vi "GetDescendants.vi"(8 "error in":errorcluster, 11 "node in":refnum<data-value>) -> (0 "error out":errorcluster, 3 "descendants":refnum<data-value>[](array[refnum]))   [LabVIEW 2023, in "CEF.lvlib" / "CEF_Node.lvclass"]
doc: "Copyright 2017 National Instruments Corporation\n\nLicensed under the Apache License, Version 2.0 (the \"License\"); you may not use this file except in compliance with the License. You may obtain a copy of the License at http://www.apache.org/licenses/LICENSE-2.0\nUnless required by applicable law or agreed to in writing, software distributed under the License is distributed on an \"AS IS\" BASIS, WITHOUT WARRANTIES OR CONDITIONS OF ANY KIND, either express or implied. See the License for the specific language governing permissions and limitations under the License."
uses:
  CEF_Node.lvclass
  CEF_Node.lvclass/CEF_Node.ctl
  ReadChildren.vi
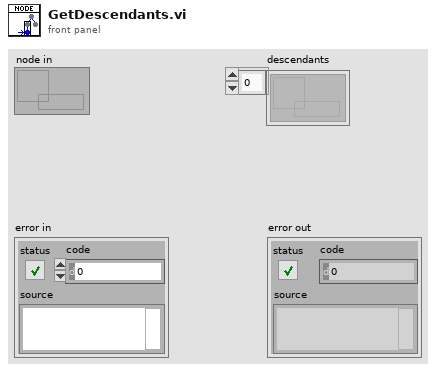
[diagram p1: front panel]
types:
  T1 = typedef "CEF.lvlib/CEF_Node.lvclass/NodeRef.ctl" = refnum<data-value>
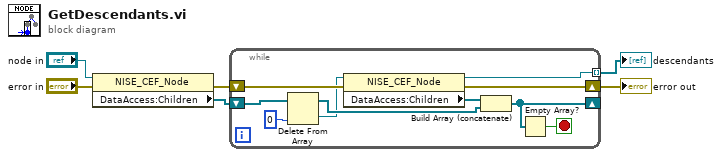
[diagram p0: block diagram]
diagram:
  n1 = property class="NISE_CEF_Node"(reference="node in", error in="error in") -> (error out=w3:errorcluster, "DataAccess:Children"=w4:T1[])  [unwired: 1 out]
  n2 = while {
    shift-right: [w9] -> _
    shift-left: w4 -> [w16]
    shift-right: [w13] -> w2
    shift-left: w3 -> [w14]
    tunnel: [w7] -> w1 mode=indexing
    stop <- w8 stop-if-true
    n3 = Delete From Array(array=w16, index=0) -> (deleted portion=w11:T1, array with subset deleted=w12:T1[])  [unwired: 1 in]
    n4 = property class="NISE_CEF_Node"(reference=w11, error in=w14) -> (reference out=w7:T1, error out=w13:errorcluster, "DataAccess:Children"=w10:T1[])
    n5 = Build Array (concatenate)(w10, w12) -> (w9:T1[])
    n6 = Empty Array?(array=w9) -> (empty?=w8:bool)
  }
  "error out" <- w2
  "descendants" <- w1
